vi "Init Slider Boundaries.vi"(11 "DofType":T1) -> (1 "Unit Labels":string[](array[string]), 2 "Dof Labels":string[](array[string]), 3 "Boundaries":cluster{"[0]":dbl, "[1]":dbl}[](array[cluster]))   [LabVIEW 2009]
uses:
  Data Access Objects/Limits/DofTypes.ctl
  Data Access Objects/Metadata/Persistant DAO Actions.ctl
panel:
  in  "Cart Displacement Labels":string[](array[string])=["Displacement X", "Displacement Y", "Displacement Z", "Rotation X", "Rotation Y", "Rotation Z"]
  in  "Cart Force Labels":string[](array[string])=["Force X", "Force Y", "Force Z", "Moment X", "Moment Y", "Moment Z"]
  in  "Act Force Labels":string[](array[string])=["Force X1", "Force X2", "Force Y1", "Force Z1", "Force Z2", "Force Z3"]
  in  "Act Disp Labels":string[](array[string])=["Displacement X1", "Displacement X2", "Displacement Y1", "Displacement Z1", "Displacement Z2", "Displacement Z3"]
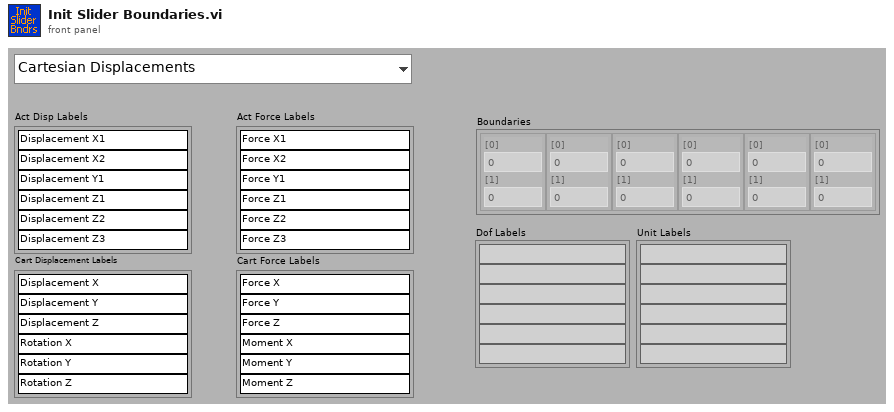
[diagram p1: front panel]
types:
  T1 = typedef "DofTypes.ctl" = enum16{"Cartesian Displacements", "Cartesian Forces & Moments", "Actuator Displacements", "Actuator Forces"}
  T2 = typedef "Persistant DAO Actions.ctl" = enum16{"Init", "Get", "Set", "Load", "Save"}
  T3 = typedef "Limit Boundary Parameters.ctl" = cluster{"Lower":dbl, "Upper":dbl, "Label":string}
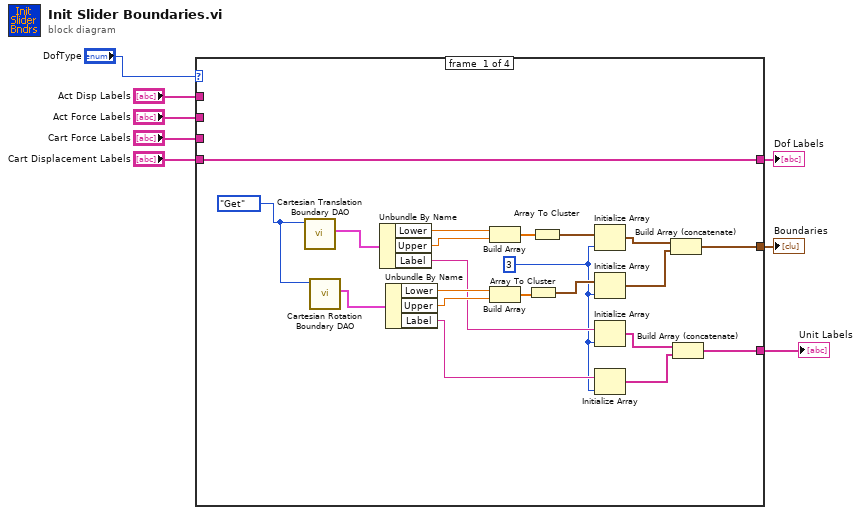
[diagram p0: block diagram]
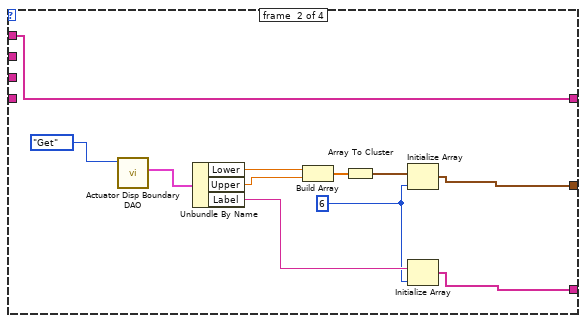
[diagram p2: hidden frame]
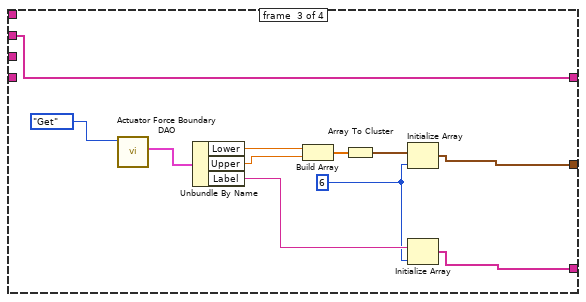
[diagram p3: hidden frame]
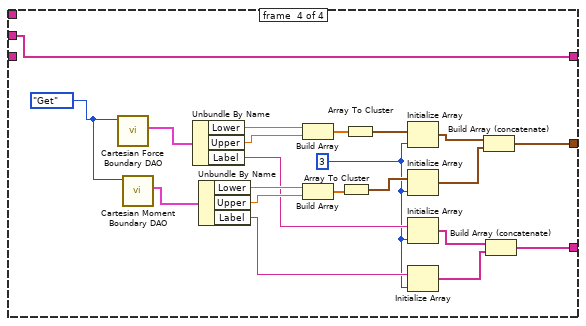
[diagram p4: hidden frame]
diagram:
  n1 = case shown="\"Cartesian Forces & Moments\"" "DofType" {
    tunnel: "Act Disp Labels" -> [_ w30 _ _]
    tunnel: "Act Force Labels" -> [_ _ w41 _]
    tunnel: "Cart Force Labels" -> [_ _ _ w52]
    tunnel: "Cart Displacement Labels" -> [w9 _ _ _]
    tunnel: [w13 w31 w42 w56] -> w1
    tunnel: [w10 w32 w43 w53] -> w2
    tunnel: [w9 w30 w41 w52] -> w3
    frame #0 {
      w16 = 3 ("dimension size")
      w29 = Persistant_DAO_Actions."Get" ("Actions")
      n2 = call "Cartesian Translation Boundary DAO.vi"("Actions"=w29) -> ("Limit Boundary Parameters Out"=w28:T3)  [unwired: 8 in, 2 out]
      n3 = call "Cartesian Rotation Boundary DAO.vi"("Actions"=w29) -> ("Limit Boundary Parameters Out"=w27:T3)  [unwired: 8 in, 2 out]
      n4 = Unbundle By Name(w28) -> ("Lower"=w26:dbl, "Upper"=w25:dbl, "Label"=w18:string)
      n5 = Unbundle By Name(w27) -> ("Lower"=w24:dbl, "Upper"=w23:dbl, "Label"=w17:string)
      n6 = Build Array(w26, w25) -> (w22:dbl[])
      n7 = Build Array(w24, w23) -> (w20:dbl[])
      n8 = Array To Cluster(array=w20) -> (cluster=w19:cluster{"[0]":dbl, "[1]":dbl})
      n9 = Array To Cluster(array=w22) -> (cluster=w21:cluster{"[0]":dbl, "[1]":dbl})
      n10 = Initialize Array(w21, w16) -> (w15:cluster{"[0]":dbl, "[1]":dbl}[])
      n11 = Initialize Array(w19, w16) -> (w14:cluster{"[0]":dbl, "[1]":dbl}[])
      n12 = Initialize Array(w18, w16) -> (w12:string[])
      n13 = Initialize Array(w17, w16) -> (w11:string[])
      n14 = Build Array (concatenate)(w15, w14) -> (w13:cluster{"[0]":dbl, "[1]":dbl}[])
      n15 = Build Array (concatenate)(w12, w11) -> (w10:string[])
    }
    frame #1 {
      w33 = 6 ("dimension size")
      n16 = call "Actuator Disp Boundary DAO.vi"("Actions"=Persistant_DAO_Actions."Get") -> ("Limit Boundary Parameters Out"=w39:T3)  [unwired: 8 in, 2 out]
      n17 = Unbundle By Name(w39) -> ("Lower"=w38:dbl, "Upper"=w37:dbl, "Label"=w34:string)
      n18 = Build Array(w38, w37) -> (w36:dbl[])
      n19 = Array To Cluster(array=w36) -> (cluster=w35:cluster{"[0]":dbl, "[1]":dbl})
      n20 = Initialize Array(w35, w33) -> (w31:cluster{"[0]":dbl, "[1]":dbl}[])
      n21 = Initialize Array(w34, w33) -> (w32:string[])
    }
    frame #2 {
      w44 = 6 ("dimension size")
      n22 = call "Actuator Force Boundary DAO.vi"("Actions"=Persistant_DAO_Actions."Get") -> ("Limit Boundary Parameters Out"=w50:T3)  [unwired: 8 in, 2 out]
      n23 = Unbundle By Name(w50) -> ("Lower"=w49:dbl, "Upper"=w48:dbl, "Label"=w45:string)
      n24 = Build Array(w49, w48) -> (w47:dbl[])
      n25 = Array To Cluster(array=w47) -> (cluster=w46:cluster{"[0]":dbl, "[1]":dbl})
      n26 = Initialize Array(w46, w44) -> (w42:cluster{"[0]":dbl, "[1]":dbl}[])
      n27 = Initialize Array(w45, w44) -> (w43:string[])
    }
    frame #3 {
      w59 = 3 ("dimension size")
      w72 = Persistant_DAO_Actions."Get" ("Actions")
      n28 = call "Cartesian Force Boundary DAO.vi"("Actions"=w72) -> ("Limit Boundary Parameters Out"=w71:T3)  [unwired: 8 in, 2 out]
      n29 = call "Cartesian Moment Boundary DAO.vi"("Actions"=w72) -> ("Limit Boundary Parameters Out"=w70:T3)  [unwired: 8 in, 2 out]
      n30 = Unbundle By Name(w71) -> ("Lower"=w69:dbl, "Upper"=w68:dbl, "Label"=w61:string)
      n31 = Unbundle By Name(w70) -> ("Lower"=w67:dbl, "Upper"=w66:dbl, "Label"=w60:string)
      n32 = Build Array(w69, w68) -> (w65:dbl[])
      n33 = Build Array(w67, w66) -> (w63:dbl[])
      n34 = Array To Cluster(array=w63) -> (cluster=w62:cluster{"[0]":dbl, "[1]":dbl})
      n35 = Array To Cluster(array=w65) -> (cluster=w64:cluster{"[0]":dbl, "[1]":dbl})
      n36 = Initialize Array(w64, w59) -> (w58:cluster{"[0]":dbl, "[1]":dbl}[])
      n37 = Initialize Array(w62, w59) -> (w57:cluster{"[0]":dbl, "[1]":dbl}[])
      n38 = Initialize Array(w61, w59) -> (w55:string[])
      n39 = Initialize Array(w60, w59) -> (w54:string[])
      n40 = Build Array (concatenate)(w58, w57) -> (w56:cluster{"[0]":dbl, "[1]":dbl}[])
      n41 = Build Array (concatenate)(w55, w54) -> (w53:string[])
    }
  }
  "Dof Labels" <- w3
  "Unit Labels" <- w2
  "Boundaries" <- w1
